vi "LPF.vi"() -> ()   [LabVIEW 2014]
uses:
  <vilib>/Analysis/2dsp.llb/Real FFT.vi
  <vilib>/Analysis/3filter.llb/Butterworth Filter (DBL).vi
  <vilib>/Analysis/NI_AALBase.lvlib
  <vilib>/Analysis/NI_AALPro.lvlib
panel:
  in  "停止":bool
  in  "阶数":i32(slide)=4 caption="滤波器阶数" scale=0.0..10.0
  in  "截止频率":dbl(slide)=20.0 caption="低截止频率:fl" scale=0.0..50.0
  in  "信号频率":dbl=20.0 format="%.2f"
  in  "采样频率":dbl=1000.0
  in  "samples":i32=500 caption="采样数"
  out "滤波后信号频谱":dbl[](graph)
  out "输入信号频谱":dbl[](graph)
  out "滤波后信号":dbl[](graph)
  out "输入信号":dbl[](graph)
  # "基于labview的低通滤波器"
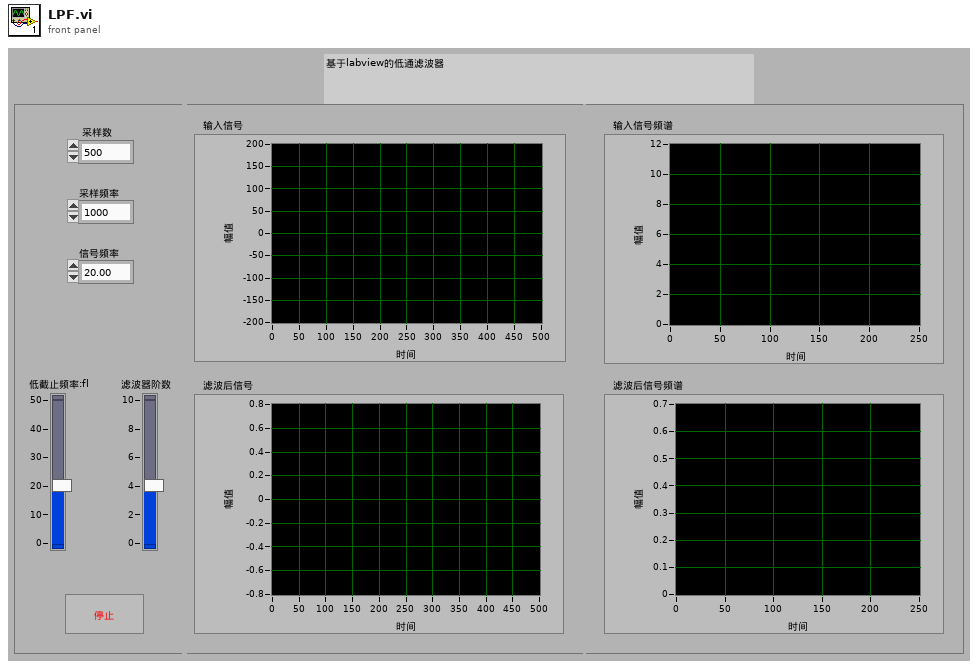
[diagram p1: front panel]
types:
  T1 = enum32{"Lowpass", "Highpass", "Bandpass", "Bandstop"}
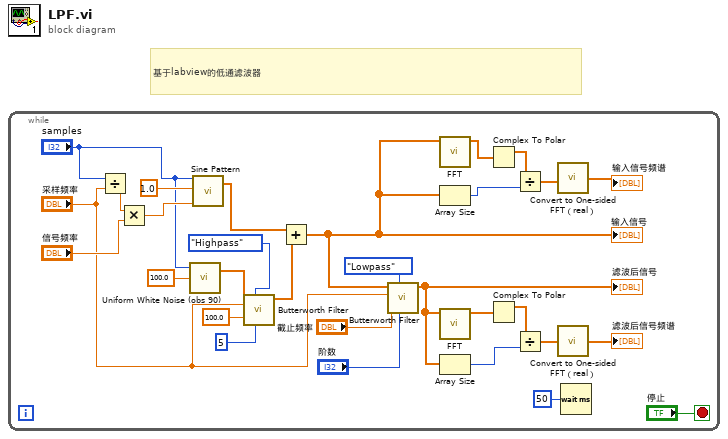
[diagram p0: block diagram]
diagram:
  # "基于labview的低通滤波器"
  n1 = while {
    stop <- "停止" stop-if-true
    n2 = Divide(x="samples", y="采样频率") -> (x/y=w29:dbl)
    n3 = Multiply(x=w29, y="信号频率") -> (x*y=w27:dbl)
    n4 = call <vilib>:"Uniform White Noise (obs 90).vi"("amplitude"=100.0, "samples"="samples") -> ("uniform white noise"=w24:dbl[])  [unwired: 1 in, 1 out]
    n5 = call <vilib>:"Sine Pattern.vi"("cycles"=w27, "amplitude"=1.0, "samples"="samples") -> ("Sinusoidal Pattern"=w21:dbl[])  [unwired: 1 in, 1 out]
    n6 = call-poly <vilib>:"Butterworth Filter.vi"("order"=5, "filter type"=T1."Highpass", "low cutoff freq: fl"=100.0, "sampling freq: fs"="采样频率", "X"=w24) -> ("Filtered X"=w20:dbl[])  [unwired: 3 in, 1 out]
    n7 = Add(x=w21, y=w20) -> (x+y=w3:dbl[])
    "输入信号" <- w3
    n8 = call-poly <vilib>:"Butterworth Filter.vi"("order"="阶数", "filter type"=T1."Lowpass", "low cutoff freq: fl"="截止频率", "sampling freq: fs"="采样频率", "X"=w3) -> ("Filtered X"=w17:dbl[])  [unwired: 3 in, 1 out]
    "滤波后信号" <- w17
    n9 = call-poly <vilib>:"FFT.vi"("X"=w3) -> ("FFT {X}"=w10:cdb[])  [unwired: 9 in, 1 out]
    n10 = Array Size(array=w3) -> (size(s)=w11:i32)
    n11 = call-poly <vilib>:"FFT.vi"("X"=w17) -> ("FFT {X}"=w16:cdb[])  [unwired: 9 in, 1 out]
    n12 = Array Size(array=w17) -> (size(s)=w14:i32)
    n13 = Complex To Polar(r * e^(i*theta)=w10) -> (r=w9:dbl[])  [unwired: 1 out]
    n14 = Complex To Polar(r * e^(i*theta)=w16) -> (r=w15:dbl[])  [unwired: 1 out]
    n15 = Divide(x=w9, y=w11) -> (x/y=w8:dbl[])
    n16 = Divide(x=w15, y=w14) -> (x/y=w13:dbl[])
    n17 = call "Convert to One-sided FFT（real）.vi"("two-sided spectrum (real)"=w8) -> ("one-sided spectrum (real)"=→"输入信号频谱":dbl[])
    n18 = call "Convert to One-sided FFT（real）.vi"("two-sided spectrum (real)"=w13) -> ("one-sided spectrum (real)"=→"滤波后信号频谱":dbl[])
    n19 = Wait (ms)(milliseconds to wait=u32 50 ("等待时间（毫秒）")) -> ()  [unwired: 1 out]
  }
